vi "Sub Super Duper_2014 05 30_JWa.vi"(0 "VISA resource name":refnum<visa-resource-name>="GPIB0::17::INSTR", 1 "Sample Properties:":T9 {"Date Created" format="%<%Y/%m/%d>T"}, 2 "Gated SMU4 is...":bool, 3 "TRF Cluster":T10={"Step 4"=-38.0, "# of Loops"=1.0, "Transfer 2"=FALSE, "Start 4"=-2.0, "Total Points 2"=2, "Start 3"=40.0, "Stop 2"=-40.0, "Step 3"=-1.0, "Loop Step"=0.0, "Integration Time 3"=0, "Loop Wait"=0.0, "First Step"=0.0} {"Loop Wait" format="%<%H:%M:%S>t"; "Integration Time 3" scale=0.0..2.0; "Step 3" format="%.2f"; "Stop 2" format="%.2f"; "Start 3" format="%.2f"; "Start 4" format="%.2f"; "Step 4" format="%.2f"}, 4 "TSP Cluster":T11={"Transport"=FALSE, "Start 2"=0.0, "Stop 3"=-60.0, "Step 2"=-1.0, "Start"=0.0, "Step"=-10.0, "Total Points"=7, "Integration Time"=0} {"Integration Time" scale=0.0..2.0; "Step" format="%.2f"; "Start" format="%.2f"; "Step 2" format="%.2f"; "Stop 3" format="%.2f"; "Start 2" format="%.2f"}, 5 "Compliance Cluster":T6={"Var1 sweep settings"={"sweep spacing (linear: 0)"=0, "sweep mode"=FALSE, "compliance (V)"=100.0, "compliance (A)"=0.001}, "Var1 sweep settings 2"={"sweep spacing (linear: 0)"=0, "sweep mode"=FALSE, "compliance (V)"=100.0, "compliance (A)"=0.001}, "Var2 step settings 2"={"compliance (A)"=0.001, "compliance (V)"=100.0}, "Var2 step settings"={"compliance (A)"=0.001, "compliance (V)"=100.0}} {"Var2 step settings"."compliance (V)" format="%.2f"; "Var2 step settings"."compliance (A)" format="%^.2e"; "Var2 step settings 2"."compliance (V)" format="%.2f"; "Var2 step settings 2"."compliance (A)" format="%^.2e"; "Var1 sweep settings 2"."compliance (A)" format="%^.2e"; "Var1 sweep settings 2"."compliance (V)" format="%.2f"; "Var1 sweep settings 2"."sweep spacing (linear: 0)" items=["linear", "log 10", "log 25", "log 50"]; "Var1 sweep settings"."compliance (A)" format="%^.2e"; "Var1 sweep settings"."compliance (V)" format="%.2f"; "Var1 sweep settings"."sweep spacing (linear: 0)" items=["linear", "log 10", "log 25", "log 50"]}, 6 "Light Bathe Cluster":T2={"TG to BG:  "=FALSE, "TG to BG Durration"=120.0, "TRF to TSP:   "=FALSE, "TRF to TSP Duration"=120.0, "Post Measure: "=FALSE, "TG to BG (TSP):"=FALSE, "TG to BG Durration 3"=120.0} {"TG to BG Durration 3" format="%<%H:%M:%S>t"; "TRF to TSP Duration" format="%<%H:%M:%S>t"; "TG to BG Durration" format="%<%H:%M:%S>t"}, 7 "error in":errorcluster, 8 "Saved Folder:":path=path "C:/1DATA/2011", 9 "Wait Cluster":T5 {"Wait Time (s)" format="%.1g"; "Wait Countdown" format="%<%H:%M:%S%1u>t"}, 11 "TG Dielectric Prop":T1, 13 "Stop \nCountdown":bool, 15 "Loop Count":dbl, 16 "Gate Current Cluster":T3={"Gate Current (TSP)"={"Y2 axis on/off"=FALSE, "MINIMUM"=0.0, "MAXIMUM"=1.0, "Variable name"="Ig", "LIN or LOG axis"="LIN"}, "Gate Current (TRF)"={"Y2 axis on/off"=FALSE, "MINIMUM"=0.0, "MAXIMUM"=1.0, "Variable name"="Ig", "LIN or LOG axis"="LIN"}} {"Gate Current (TSP)"."MAXIMUM" format="%.9f"; "Gate Current (TSP)"."MINIMUM" format="%.9f"; "Gate Current (TRF)"."MAXIMUM" format="%.9f"; "Gate Current (TRF)"."MINIMUM" format="%.9f"}, 17 "Dielectric Constant (BG)":dbl) -> (12 "Status Indicator":bool, 14 "Vt Cluster":T4 {"Id Max" format="%.3g"; "Vt Max" format="%.3g"; "Vt Min" format="%.3g"; "Vt Ratio" format="%.3g"}, 20 "VISA resource name out":refnum<visa-resource-name>, 21 "TRF Path":path, 23 "TSP Path":path, 24 "Graph Cluster":T7, 25 "Char Cluster":T8 {"Mobility-Lin" format="%#_4e"; "On/Off" format="%#_4e"; "Mobility-Sat" format="%#_4e"}, 27 "error out":errorcluster)   [LabVIEW 2012]
uses:
  <vilib>/Platform/TimedLoop/XDataNode/wakeup.ctl
  <vilib>/Platform/TimedLoop/XDataNode/XDNodeRunTimeDep.lvlib
  <vilib>/Platform/TimedLoop/XDataNode/nitl_modes.ctl
  <vilib>/Platform/TimedLoop/XDataNode/timing_clust.ctl
  <vilib>/Platform/TimedLoop/XDataNode/XDataNode.xnode
panel:
  in  "Ambient Temp (Y/N)":bool=TRUE
  out "LKG Path":path
  # "Vg Sweep"
  # "Vd Step"
  # "Loops and Integration Time"
  # "Device Characteristics"
  # "Light Bath is..."
  # "Duration (hh:mm:ss)"
  # "Sample Properties:"
  # "%"
  # "nm"
  # "Device Properties:"
  # "um"
  # "um"
  # "Vg Step"
  # "Vd Step"
  # "Integration Time"
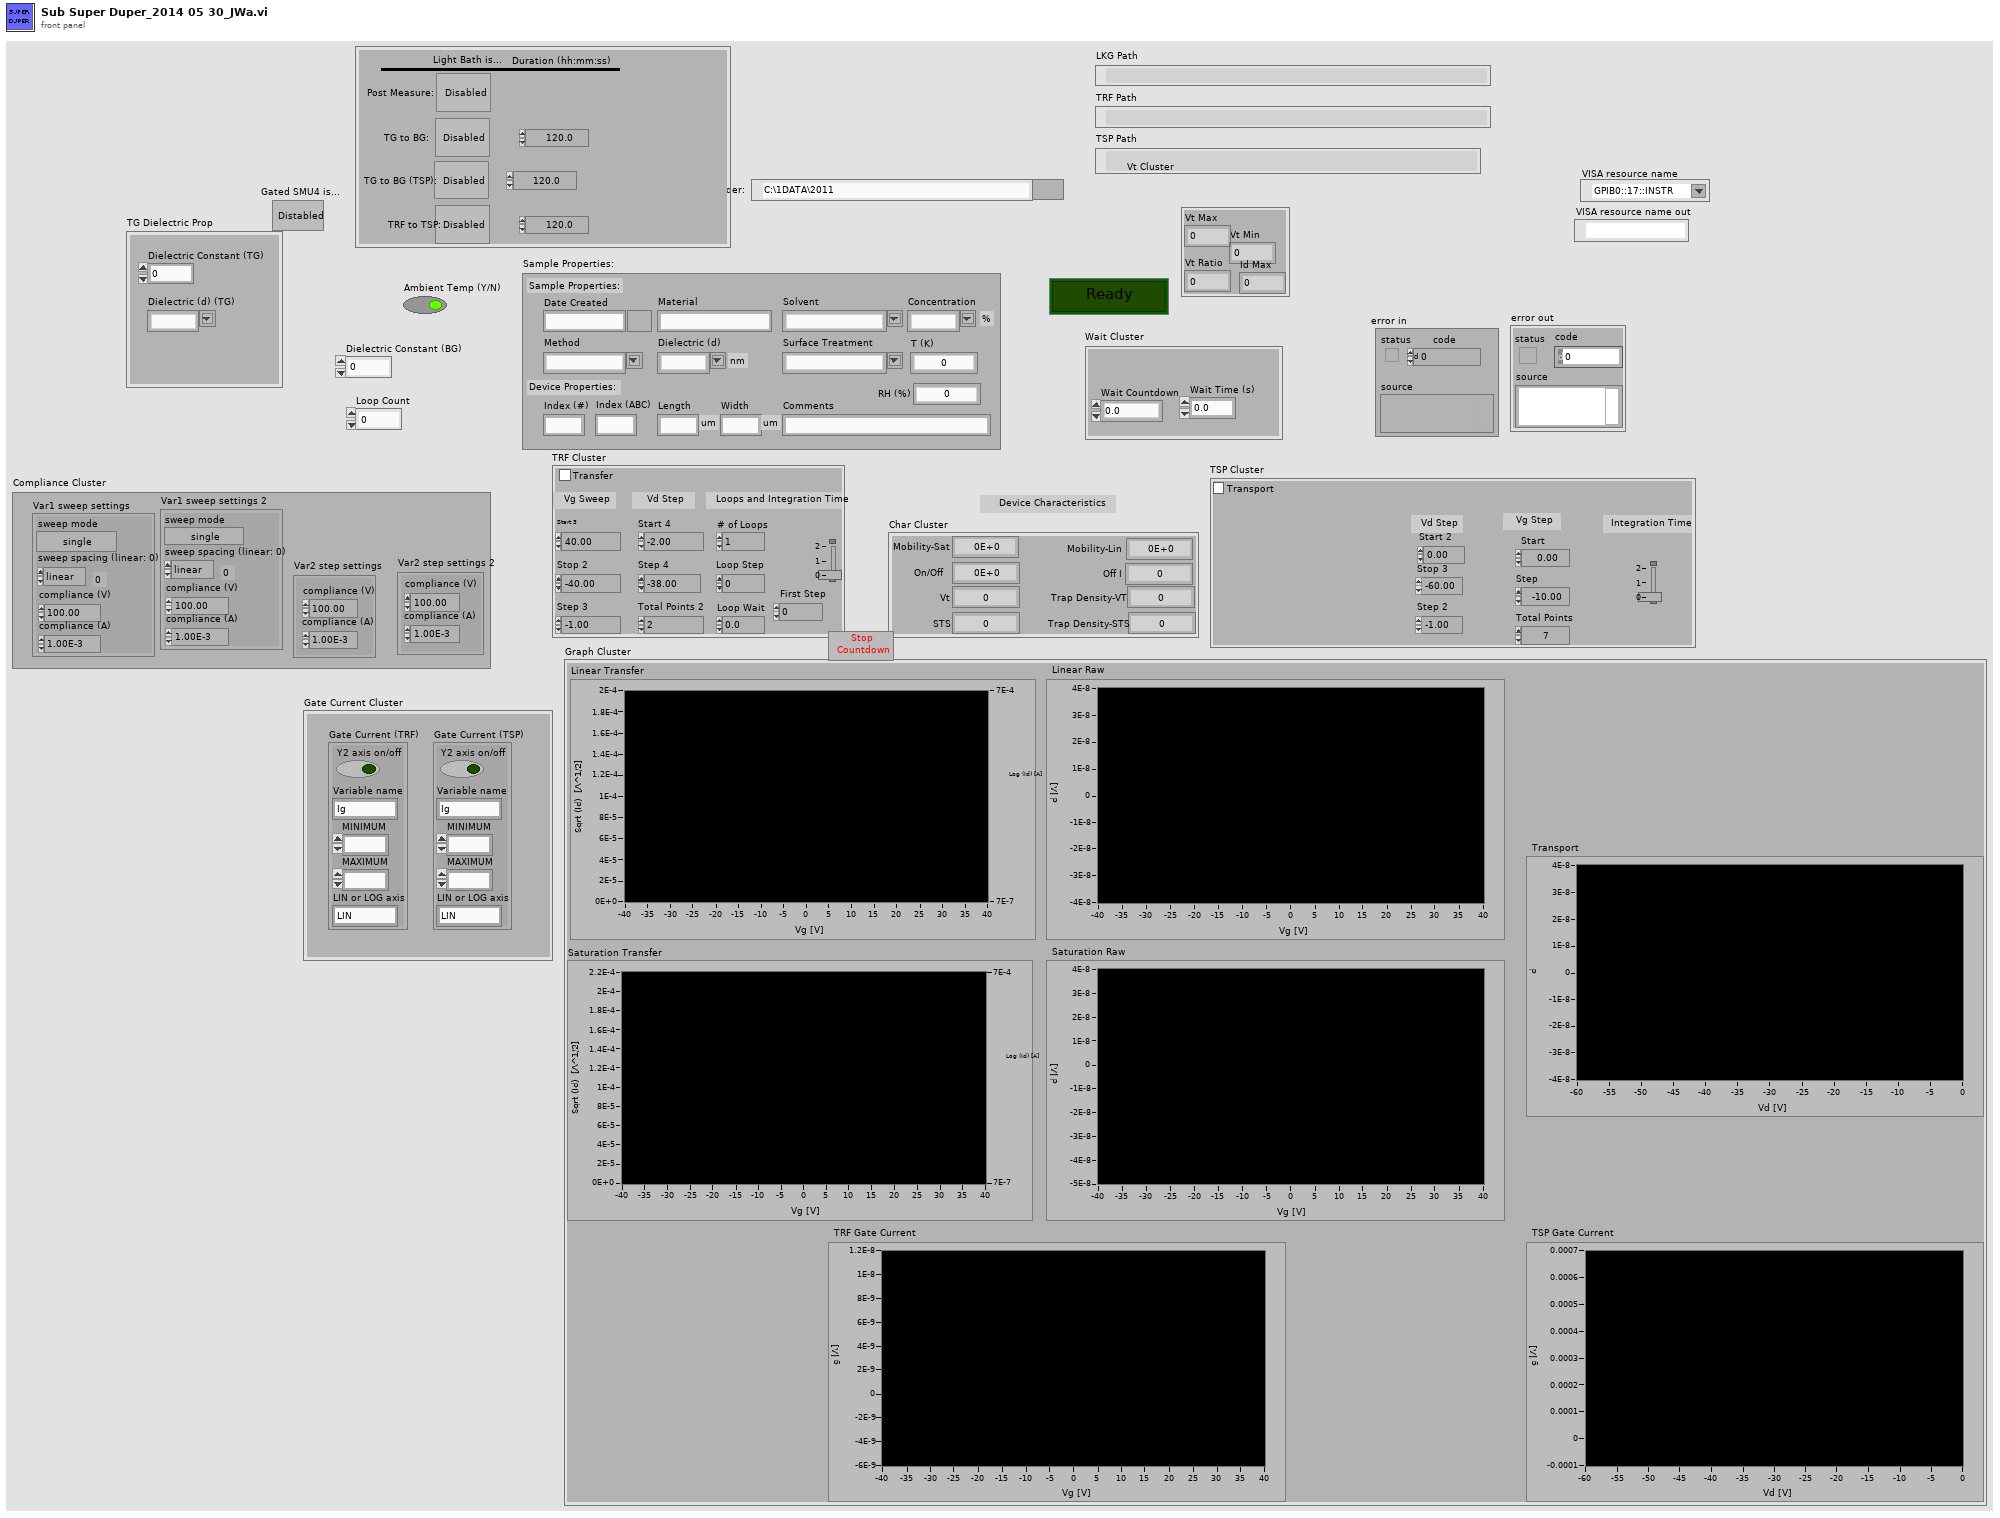
[diagram p1: front panel]
types:
  T1 = cluster{"Dielectric Constant (TG)":dbl, "Dielectric (d) (TG)":string}
  T2 = cluster{"TG to BG:  ":bool, "TG to BG Durration":dbl, "TRF to TSP:   ":bool, "TRF to TSP Duration":dbl, "Post Measure: ":bool, "TG to BG (TSP):":bool, "TG to BG Durration 3":dbl}
  T3 = cluster{"Gate Current (TSP)":cluster{"Y2 axis on/off":bool, "MINIMUM":ext, "MAXIMUM":ext, "Variable name":string, "LIN or LOG axis":string}, "Gate Current (TRF)":cluster{"Y2 axis on/off":bool, "MINIMUM":ext, "MAXIMUM":ext, "Variable name":string, "LIN or LOG axis":string}}
  T4 = cluster{"Vt Max":i32, "Vt Min":i32, "Vt Ratio":i32, "Id Max":i32}
  T5 = cluster{"Wait Countdown":dbl, "Wait Time (s)":dbl}
  T6 = cluster{"Var1 sweep settings":cluster{"sweep spacing (linear: 0)":u16, "sweep mode":bool, "compliance (V)":dbl, "compliance (A)":dbl}, "Var1 sweep settings 2":cluster{"sweep spacing (linear: 0)":u16, "sweep mode":bool, "compliance (V)":dbl, "compliance (A)":dbl}, "Var2 step settings 2":cluster{"compliance (A)":dbl, "compliance (V)":dbl}, "Var2 step settings":cluster{"compliance (A)":dbl, "compliance (V)":dbl}}
  T7 = cluster{"Linear Transfer":cluster{dbl[], "trace":dbl[]}[], "Linear Raw":cluster{dbl[], dbl[]}[], "Saturation Transfer":cluster{dbl[], "trace":dbl[]}[], "Saturation Raw":cluster{dbl[], dbl[]}[], "Transport":cluster{dbl[], dbl[]}[], "TRF Gate Current":cluster{dbl[], dbl[]}[], "TSP Gate Current":cluster{dbl[], dbl[]}[]}
  T8 = cluster{"Mobility-Sat":dbl, "Mobility-Lin":dbl, "On/Off ":dbl, "Off I":dbl, "Vt":dbl, "STS":dbl, "Trap Density-VT":dbl, "Trap Density-STS":dbl}
  T9 = cluster{"Date Created":timestamp, "Material":string, "Solvent":string, "Concentration":string, "Method":string, "Dielectric (d)":string, "Index (#)":string, "Index (ABC)":string, "Length":string, "Width":string, "Surface Treatment":string, "Comments":string, "T (K)":dbl, "RH (%)":dbl}
  T10 = cluster{"Step 4":dbl, "# of Loops":dbl, "Transfer 2":bool, "Start 4":dbl, "Total Points 2":u16, "Start 3":dbl, "Stop 2":dbl, "Step 3":dbl, "Loop Step":dbl, "Integration Time 3":u32, "Loop Wait":dbl, "First Step":dbl}
  T11 = cluster{"Transport":bool, "Start 2":dbl, "Stop 3":dbl, "Step 2":dbl, "Start":dbl, "Step":dbl, "Total Points":u16, "Integration Time":u32}
  T12 = cluster{"Vname":string, "Vname 2":string, "Vname 3":string, "Vname 4":string, "Iname":string, "Iname 2":string, "Iname 3":string, "Iname 4":string, "Mode":u16, "Mode 2":u16, "Mode 3":u16, "Mode 4":u16, "Function":u16, "Function 2":u16, "Function 3":u16, "Function 4":u16, "Value (V or A)":dbl, "Value (Either V or A) 2":dbl, "Value (Either V or A) 3":dbl, "Value (Either V or A) 4":dbl}
  T13 = typedef "XDNodeRunTimeDep.lvlib/timing_clust.ctl" = cluster{"Expected End [f-1]":u64, "Actual End [f-1]":u64, "Finished Late? [f-1]":bool, "Expected End [i-1]":u64, "Actual End [i-1]":u64, "Finished Late? [i-1]":bool, "Expected Start [i]":u64, "Actual Start [i]":u64, "Expected Start [f]":u64, "Actual Start [f]":u64, "Source Name":string, "Structure Name":string, "Period":i64, "Deadline":i64, "Offset":i64, "Start":i64, "Priority":i32, "Timeout":i32, "Mode":T14, "Wakeup Reason":T15, "Error":errorcluster, "Source Type":string, "Secondary Source Type":string, "Global End Time":u64, "Global Start Time":u64, "Frame Duration":u64, "Iteration Duration":u64, "Assigned CPU":i32, "I/O Scan Engine Mode":u32}
  T14 = typedef "XDNodeRunTimeDep.lvlib/nitl_modes.ctl" = enum32{"No Change", "Process missed periods, maintain original phase", "Discard missed periods, maintain original phase", "Process missed periods, ignore original phase", "Discard missed periods, ignore original phase"}
  T15 = typedef "XDNodeRunTimeDep.lvlib/wakeup.ctl" = enum32{"Normal", "Aborted", "Asynchronous wakeup", "Timing source error", "Timed loop error", "Timeout"}
  T16 = cluster{"sweep spacing (linear: 0)":u16, "sweep mode":bool, "compliance (V)":dbl, "compliance (A)":dbl}
  T17 = cluster{"compliance (A)":dbl, "compliance (V)":dbl}
  T18 = cluster{"Y2 axis on/off":bool, "MINIMUM":ext, "MAXIMUM":ext, "Variable name":string, "LIN or LOG axis":string}
  T19 = cluster{"Start 3":dbl, "Stop 2":dbl, "Step 3":dbl, "sweep spacing (linear: 0)":u16, "sweep mode":bool, "compliance (V)":dbl, "compliance (A)":dbl}
  T20 = cluster{"compliance (A)":dbl, "compliance (V)":dbl, "Start 4":dbl, "Total Points 2":u16, dbl}
  T21 = cluster{"Vt Max":i32, "Vt Min":i32, "Vt Ratio":i32, "Id Max":dbl}
  T22 = cluster{"Mobility-Sat":dbl, "Mobility-Lin":dbl, "On/Off Current":dbl, "Off I":dbl, "Vt":dbl, "STS":dbl, "Trap Density-VT":dbl, "Trap Density-STS":dbl}
  T23 = cluster{"Linear Sqrt":cluster{dbl[], "trace":dbl[]}[], "Linear Log":cluster{dbl[], "trace":dbl[]}[], "Linear Raw":cluster{dbl[], dbl[]}[], "Saturation Sqrt":cluster{dbl[], "trace":dbl[]}[], "Saturation Log":cluster{dbl[], "trace":dbl[]}[], "Saturation Raw":cluster{dbl[], "trace":dbl[]}[], "Gate Current":cluster{dbl[], "trace":dbl[]}[]}
  T24 = cluster{"Start 2":dbl, "Stop 3":dbl, "Step 2":dbl, "sweep spacing (linear: 0)":u16, "sweep mode":bool, "compliance (V)":dbl, "compliance (A)":dbl}
  T25 = cluster{"compliance (A)":dbl, "compliance (V)":dbl, "Start":dbl, "Total Points":u16, "Step":dbl}
  T26 = cluster{"Transport":cluster{dbl[], dbl[]}[], "Gate Current":cluster{dbl[], dbl[]}[]}
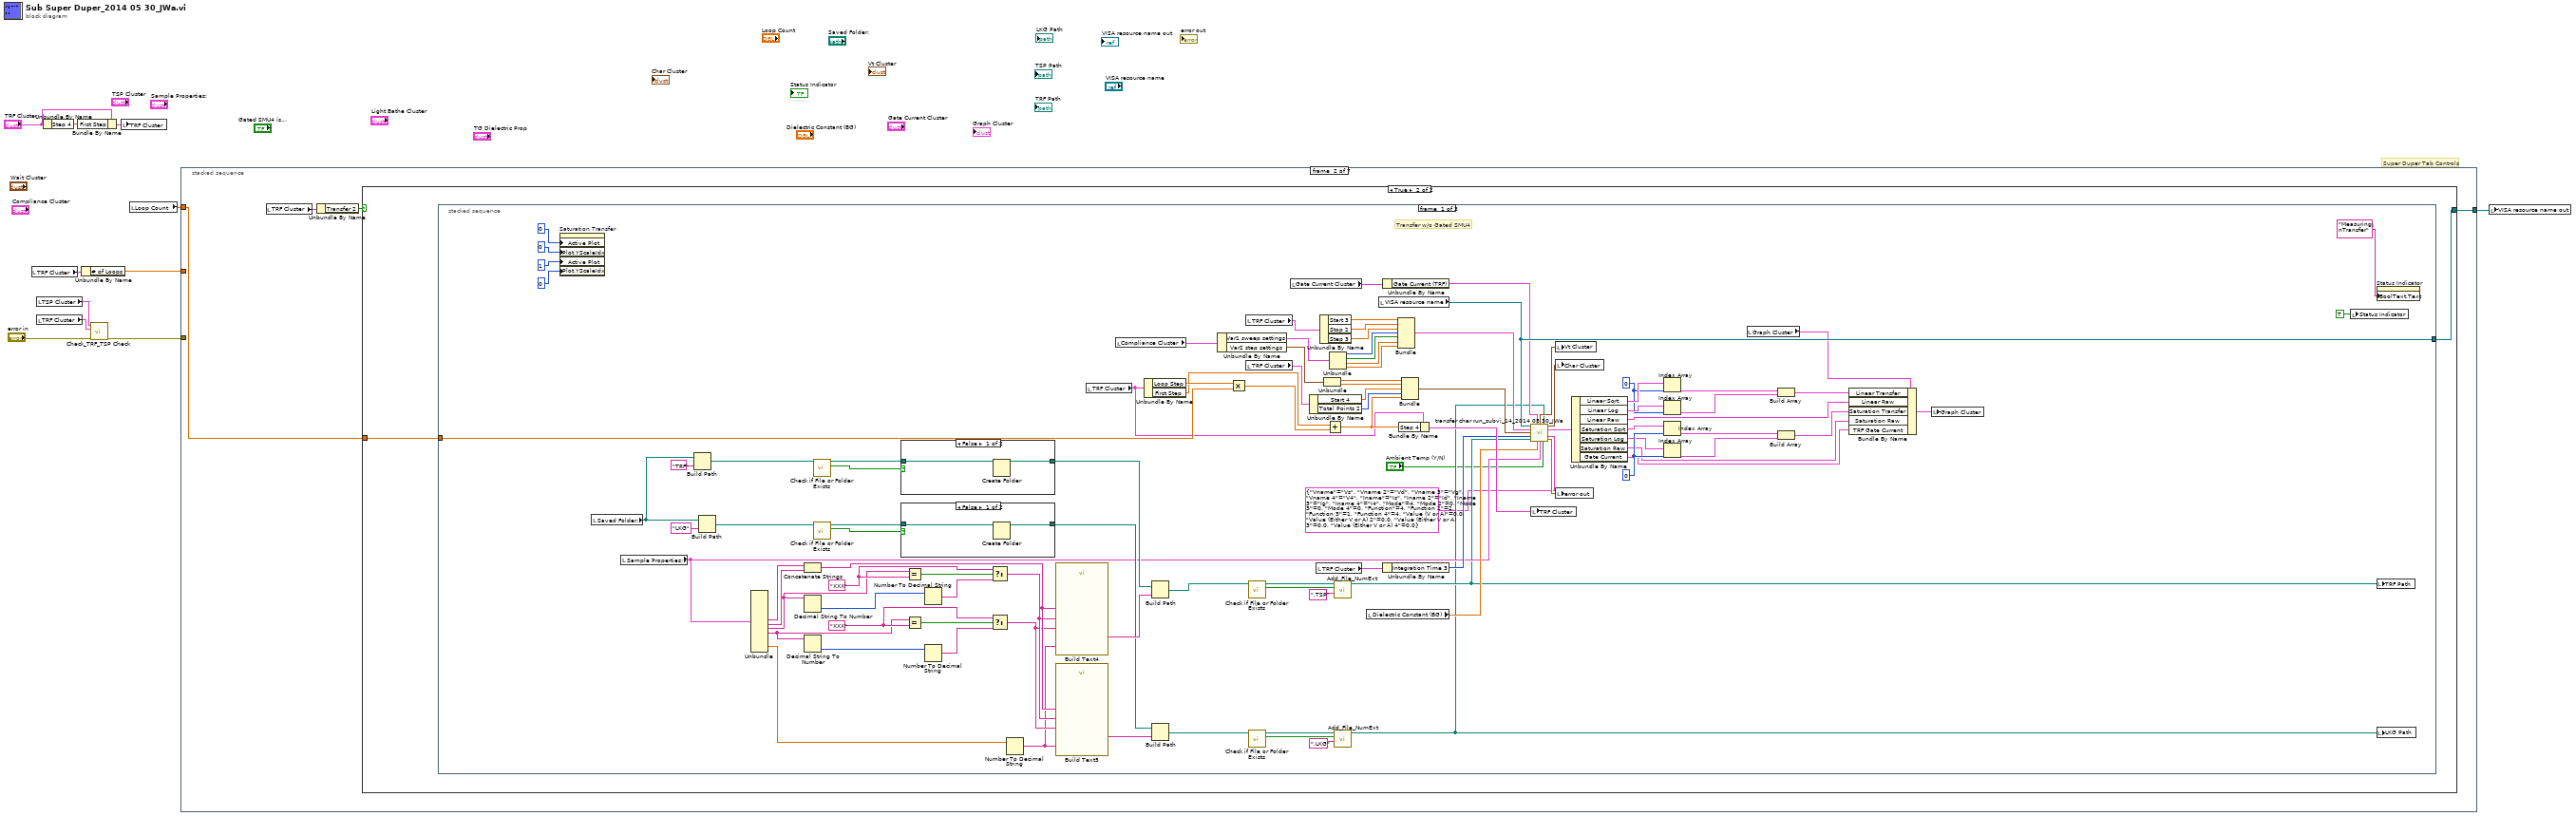
[diagram p0: block diagram]
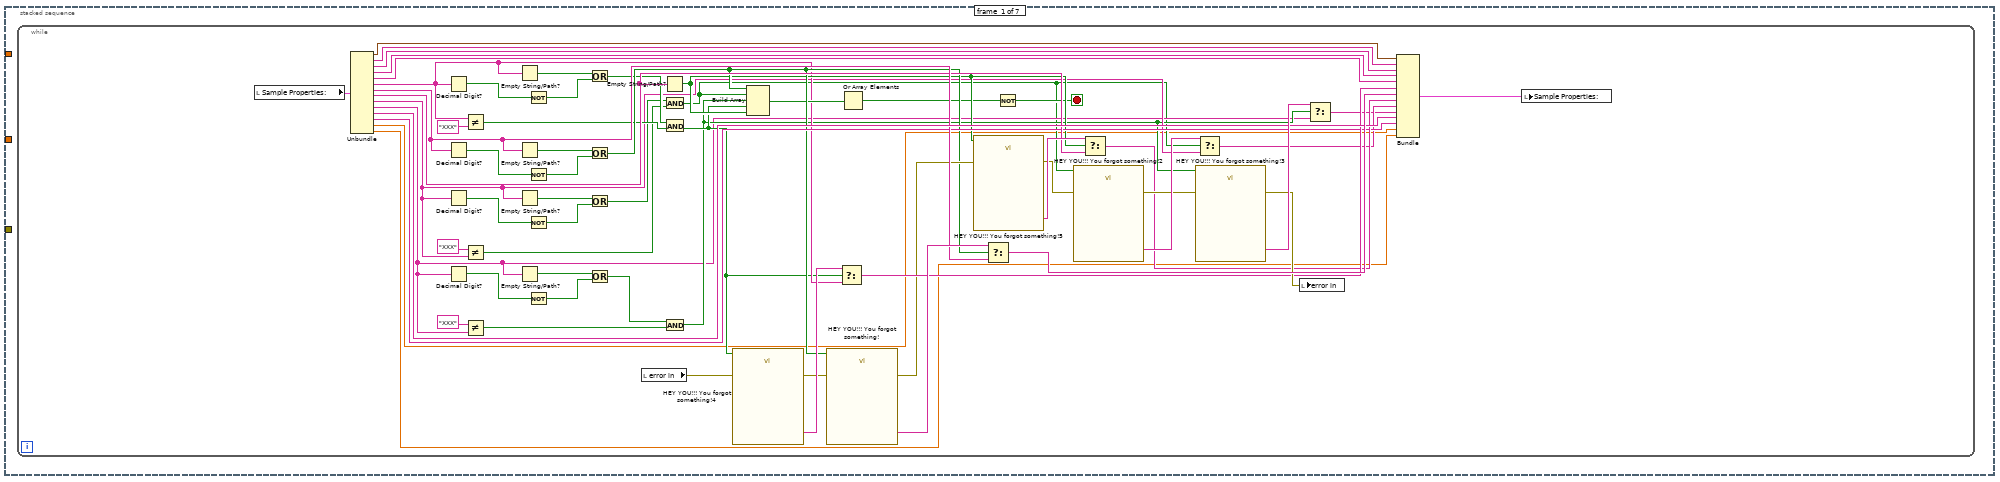
[diagram p2: hidden frame]
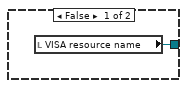
[diagram p3: hidden frame]
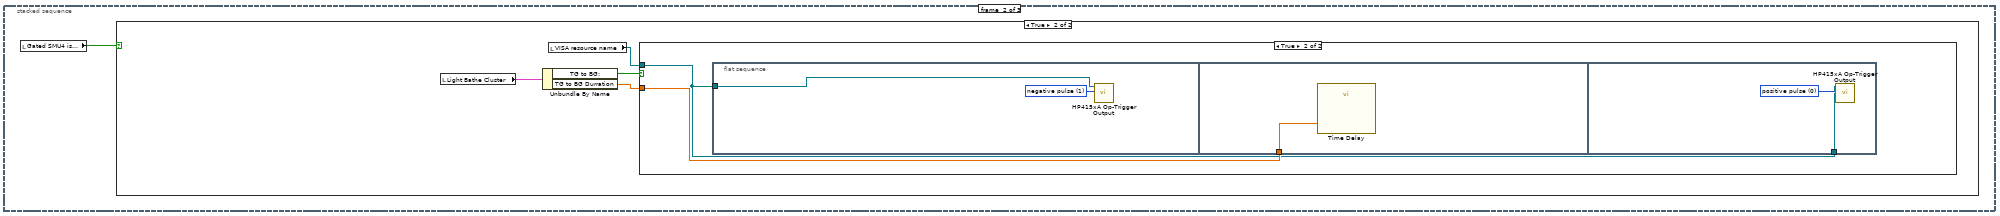
[diagram p6: hidden frame]
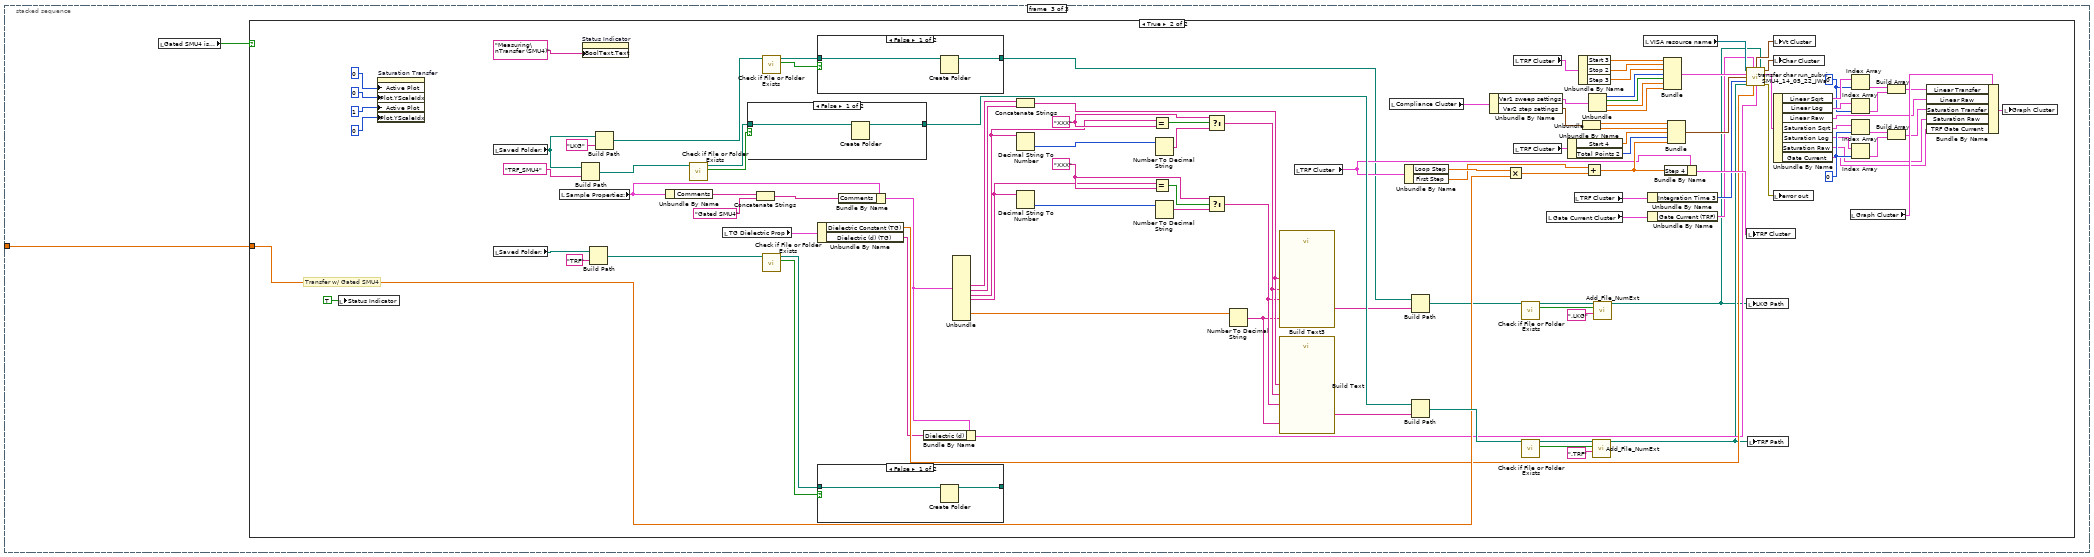
[diagram p9: hidden frame]
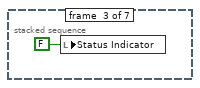
[diagram p14: hidden frame]
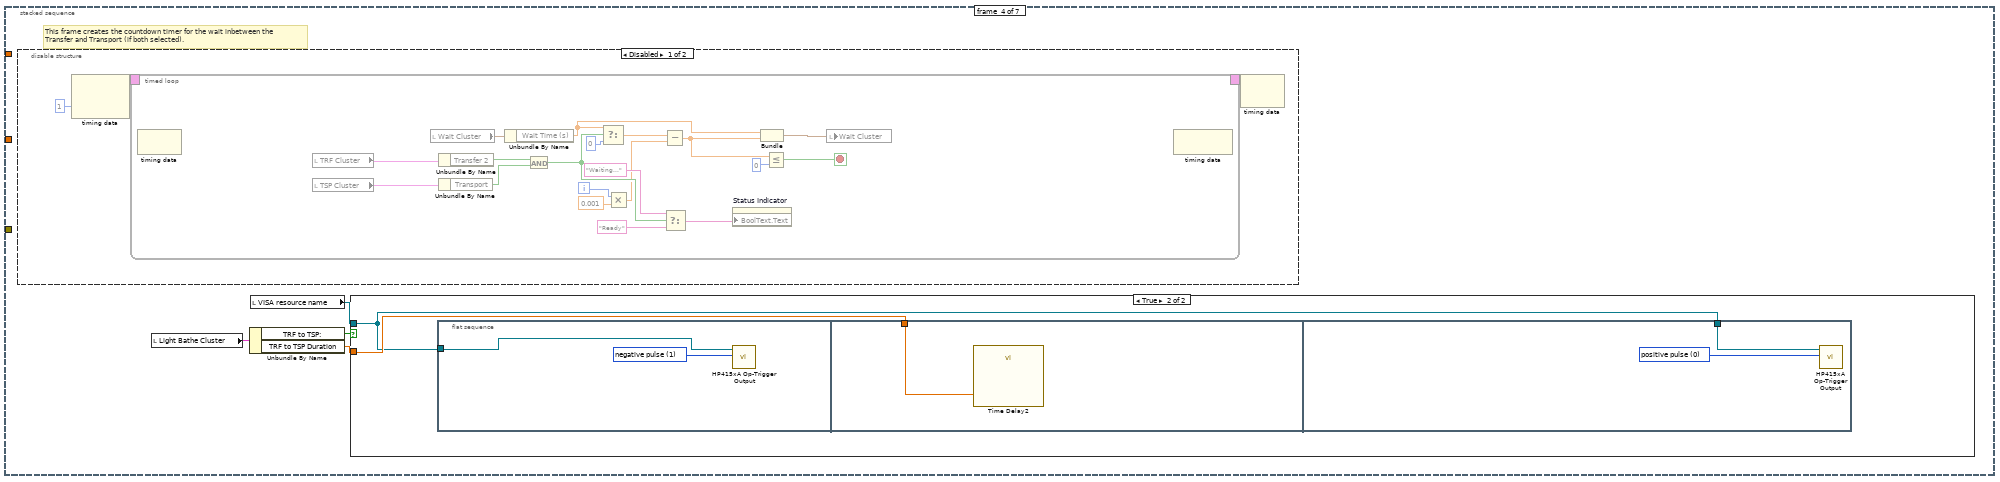
[diagram p15: hidden frame]
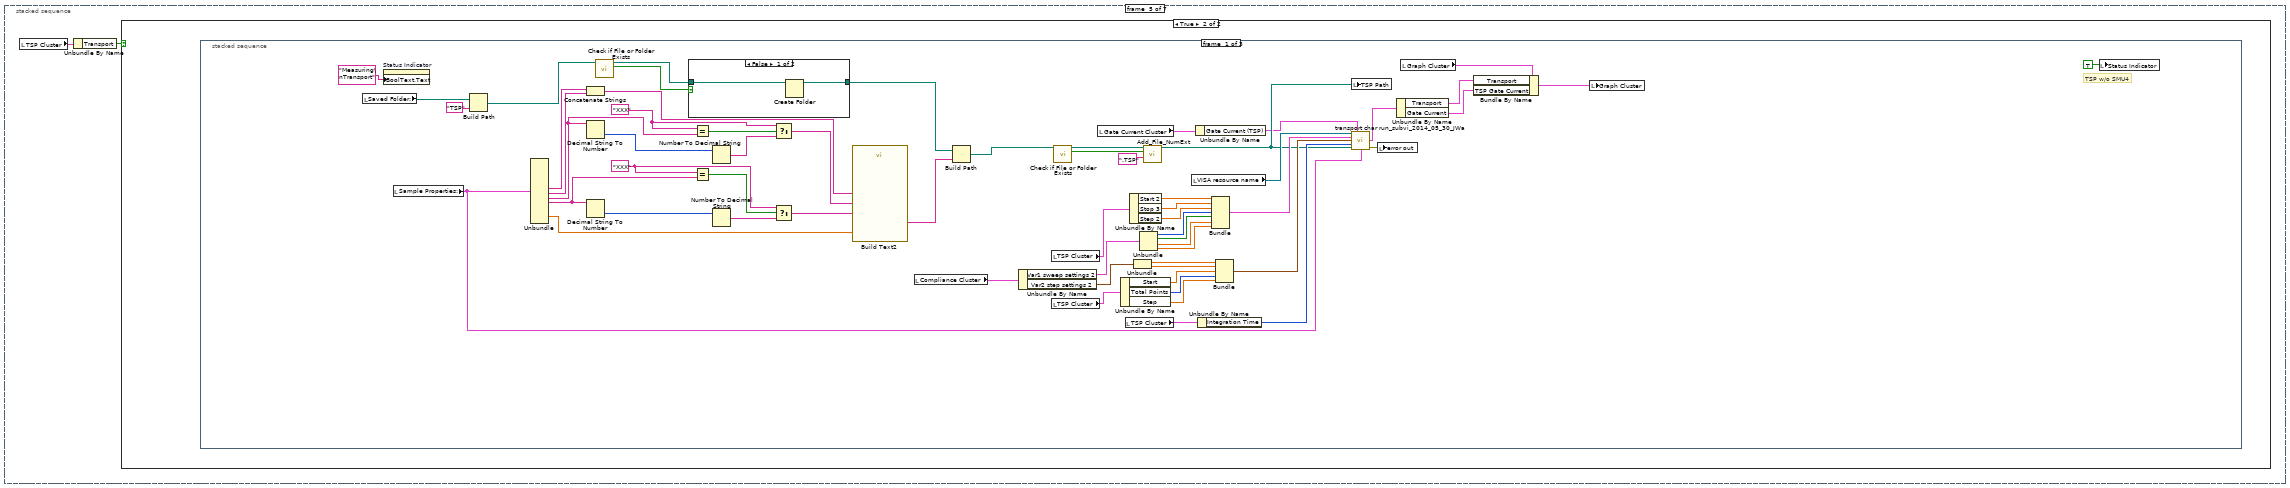
[diagram p18: hidden frame]
diagram:
  # "Super Duper Tab Controls"
  n1 = local read "TRF Cluster"() -> (w8:T10)
  n2 = local read "TSP Cluster"() -> (w4:T11)
  n3 = local read "TRF Cluster"() -> (w3:T10)
  n4 = Unbundle By Name("TRF Cluster") -> ("Step 4"=w9:dbl)
  n5 = Bundle By Name(cluster="TRF Cluster", "First Step"=w9) -> (w11:T10)
  n6 = Unbundle By Name(w8) -> ("# of Loops"=w7:dbl)
  n7 = call "Check_TRF_TSP Check.vi"("error in"="error in", "TRF Cluster"=w3, "TSP Cluster"=w4) -> ("error out"=w1:errorcluster)  [unwired: 8 in]
  n8 = local write "TRF Cluster"(w11) -> ()
  n9 = local read "Loop Count"() -> (w5:dbl)
  n10 = stacked-sequence {
    tunnel: w5 -> [_ w76 _ _ _ _ w507]
    tunnel: w7 -> [_ _ _ _ _ _ w506]
    tunnel: [_ w73 _ _ _ _ _] -> w6
    tunnel: w1 -> [_ _ _ _ _ _ _]
    frame #0 {
      n11 = while {
        stop <- w38 stop-if-true
        n12 = local read "Sample Properties:"() -> (w67:T9)
        n13 = Unbundle(w67) -> ("Date Created"=w68:timestamp, "Material"=w69:string, "Solvent"=w70:string, "Concentration"=w71:string, "Method"=w72:string, "Dielectric (d)"=w27:string, "Index (#)"=w57:string, "Index (ABC)"=w54:string, "Length"=w22:string, "Width"=w15:string, "Surface Treatment"=w60:string, "Comments"=w52:string, "T (K)"=w13:dbl, "RH (%)"=w12:dbl)
        n14 = Decimal Digit?(1:w27) -> (0:w35:bool)
        n15 = Decimal Digit?(1:w57) -> (0:w48:bool)
        n16 = Decimal Digit?(1:w22) -> (0:w37:bool)
        n17 = Decimal Digit?(1:w15) -> (0:w36:bool)
        n18 = Not Equal?(x=w27, y="XXX") -> (x != y?=w26:bool)
        n19 = Not Equal?(x="XXX", y=w22) -> (x != y?=w21:bool)
        n20 = Not Equal?(x="XXX", y=w15) -> (x != y?=w19:bool)
        n21 = Empty String/Path?(string/path=w27) -> (empty?=w29:bool)
        n22 = Empty String/Path?(string/path=w57) -> (empty?=w56:bool)
        n23 = Empty String/Path?(string/path=w22) -> (empty?=w31:bool)
        n24 = Empty String/Path?(string/path=w15) -> (empty?=w30:bool)
        n25 = Not(x=w35) -> (.not. x?=w32:bool)
        n26 = Not(x=w48) -> (.not. x?=w47:bool)
        n27 = Not(x=w37) -> (.not. x?=w34:bool)
        n28 = Not(x=w36) -> (.not. x?=w33:bool)
        n29 = Or(x=w29, y=w32) -> (x .or. y?=w25:bool)
        n30 = Or(x=w56, y=w47) -> (x .or. y?=w42:bool)
        n31 = Or(x=w31, y=w34) -> (x .or. y?=w20:bool)
        n32 = Or(x=w30, y=w33) -> (x .or. y?=w18:bool)
        n33 = local read "error in"() -> (w44:errorcluster)
        n34 = Empty String/Path?(string/path=w54) -> (empty?=w41:bool)
        n35 = And(x=w20, y=w21) -> (x .and. y?=w14:bool)
        n36 = And(x=w25, y=w26) -> (x .and. y?=w24:bool)
        n37 = And(x=w18, y=w19) -> (x .and. y?=w17:bool)
        n38 = call "HEY YOU!!! You forgot something!4"("Enable"=w24, "error in (no error)"=w44) -> ("Dielectric (d)"=w59:string, "error out"=w43:errorcluster)  [unwired: 15 in, 1 out]
        n39 = Build Array(w42, w14, w17, w24, w41) -> (w40:bool[])
        n40 = call "HEY YOU!!! You forgot something!"("Enable"=w42, "error in (no error)"=w43) -> ("Index (#)"=w66:string, "error out"=w46:errorcluster)  [unwired: 15 in, 1 out]
        n41 = Select(t=w59, s=w24, f=w27) -> (s? t:f=w58:string)
        n42 = Or Array Elements(Boolean array=w40) -> (logical OR=w39:bool)
        n43 = call "HEY YOU!!! You forgot something!5"("Enable"=w41, "error in (no error)"=w46) -> ("Index (ABC)"=w55:string, "error out"=w45:errorcluster)  [unwired: 15 in, 1 out]
        n44 = Select(t=w66, s=w42, f=w57) -> (s? t:f=w63:string)
        n45 = Not(x=w39) -> (.not. x?=w38:bool)
        n46 = call "HEY YOU!!! You forgot something!2"("Enable"=w14, "error in (no error)"=w45) -> ("Length"=w65:string, "error out"=w62:errorcluster)  [unwired: 15 in, 1 out]
        n47 = Select(t=w55, s=w41, f=w54) -> (s? t:f=w53:string)
        n48 = call "HEY YOU!!! You forgot something!3"("Enable"=w17, "error in (no error)"=w62) -> ("Width"=w64:string, "error out"=w61:errorcluster)  [unwired: 15 in, 1 out]
        n49 = Select(t=w65, s=w14, f=w22) -> (s? t:f=w51:string)
        n50 = local write "error in"(w61) -> ()
        n51 = Select(t=w64, s=w17, f=w15) -> (s? t:f=w50:string)
        n52 = Bundle("Date Created"=w68, "Material"=w69, "Solvent"=w70, "Concentration"=w71, "Method"=w72, "Dielectric (d)"=w58, "Index (#)"=w63, "Index (ABC)"=w53, "Length"=w51, "Width"=w50, "Surface Treatment"=w60, "Comments"=w52, "T (K)"=w13, "RH (%)"=w12) -> (w49:T9)  [unwired: 1 in]
        n53 = local write "Sample Properties:"(w49) -> ()
      }
    }
    frame #1 {
      n54 = local read "TRF Cluster"() -> (w74:T10)
      n55 = Unbundle By Name(w74) -> ("Transfer 2"=w75:bool)
      n56 = case shown="True" w75 {
        tunnel: w76 -> [_ w79]
        tunnel: [w77 w78] -> w73
        frame False {
          n57 = local read "VISA resource name"() -> (w77:refnum<visa-resource-name>)
        }
        frame True {
          n58 = stacked-sequence {
            tunnel: w79 -> [w180 _ w200]
            tunnel: [w179 _ _] -> w78
            frame #0 {
              w113 = 0
              w119 = 0
              w160 = "XXX"
              w163 = "XXX"
              # "Transfer w/o Gated SMU4"
              n59 = property on="Saturation Transfer" class="XYGraph (strict)"("Active Plot"=0, "Plot.YScaleIdx"=0, "Active Plot"=1, "Plot.YScaleIdx"=0) -> ()  [unwired: 2 in, 2 out]
              n60 = local read "Saved Folder:"() -> (w105:path)
              n61 = local read "Sample Properties:"() -> (w90:T9)
              n62 = Build Path(base path=w105, name or relative path="TRF") -> (appended path=w153:path)
              n63 = Build Path(base path=w105, name or relative path="LKG") -> (appended path=w101:path)
              n64 = Unbundle(w90) -> ("Index (#)"=w169:string, "Index (ABC)"=w168:string, "Length"=w157:string, "Width"=w159:string, "T (K)"=w136:dbl)  [unwired: 9 out]
              n65 = Concatenate Strings(w169, w168) -> (w98:string)
              n66 = Decimal String To Number(string=w157) -> (number=w166:i32)  [unwired: 2 in, 1 out]
              n67 = Decimal String To Number(string=w159) -> (number=w165:i32)  [unwired: 2 in, 1 out]
              n68 = call <vilib>:"Check if File or Folder Exists.vi"("path"=w153) -> ("file or folder exists?"=w155:bool, "dup path"=w154:path)  [unwired: 8 in, 1 out]
              n69 = call <vilib>:"Check if File or Folder Exists.vi"("path"=w101) -> ("file or folder exists?"=w102:bool, "dup path"=w103:path)  [unwired: 8 in, 1 out]
              n70 = case shown="False" w155 {
                tunnel: w154 -> [w185 w186]
                tunnel: [w184 w186] -> w152
                frame False {
                  n71 = Create Folder(path (use dialog)=w185) -> (created path=w184:path)  [unwired: 2 in, 2 out]
                }
                frame True {
                }
              }
              n72 = case shown="False" w102 {
                tunnel: w103 -> [w182 w183]
                tunnel: [w181 w183] -> w94
                frame False {
                  n73 = Create Folder(path (use dialog)=w182) -> (created path=w181:path)  [unwired: 2 in, 2 out]
                }
                frame True {
                }
              }
              n74 = Equal?(x=w157, y=w163) -> (x = y?=w164:bool)
              n75 = Equal?(x=w159, y=w160) -> (x = y?=w161:bool)
              n76 = Number To Decimal String(number=w166) -> (decimal integer string=w162:string)  [unwired: 1 in]
              n77 = Number To Decimal String(number=w165) -> (decimal integer string=w158:string)  [unwired: 1 in]
              n78 = Select(t=w163, s=w164, f=w162) -> (s? t:f=w97:string)
              n79 = Select(t=w160, s=w161, f=w158) -> (s? t:f=w96:string)
              n80 = Number To Decimal String(number=w136) -> (decimal integer string=w95:string)  [unwired: 1 in]
              n81 = call "Build Text4"("T"=w95, "Index"=w98, "Length"=w97, "Width"=w96) -> ("Result"=w172:string)  [unwired: 10 in, 1 out]
              n82 = call "Build Text5"("T"=w95, "Index"=w98, "Length"=w97, "Width"=w96) -> ("Result"=w99:string)  [unwired: 10 in, 1 out]
              n83 = local read "TRF Cluster"() -> (w130:T10)
              n84 = local read "Compliance Cluster"() -> (w139:T6)
              n85 = Unbundle By Name(w130) -> ("Loop Step"=w133:dbl, "First Step"=w132:dbl)
              n86 = Build Path(base path=w152, name or relative path=w172) -> (appended path=w167:path)
              n87 = Build Path(base path=w94, name or relative path=w99) -> (appended path=w100:path)
              n88 = Unbundle By Name(w139) -> ("Var1 sweep settings"=w137:T16, "Var2 step settings"=w138:T17)
              n89 = Multiply(x=w133, y=w180) -> (x*y=w135:dbl)
              n90 = local read "TRF Cluster"() -> (w144:T10)
              n91 = local read "TRF Cluster"() -> (w147:T10)
              n92 = call <vilib>:"Check if File or Folder Exists.vi"("path"=w167) -> ("file or folder exists?"=w87:bool, "dup path"=w86:path)  [unwired: 8 in, 1 out]
              n93 = call <vilib>:"Check if File or Folder Exists.vi"("path"=w100) -> ("file or folder exists?"=w82:bool, "dup path"=w83:path)  [unwired: 8 in, 1 out]
              n94 = local read "Gate Current Cluster"() -> (w93:T3)
              n95 = Unbundle By Name(w147) -> ("Start 4"=w146:dbl, "Total Points 2"=w145:u16)
              n96 = local read "TRF Cluster"() -> (w140:T10)
              n97 = Unbundle By Name(w144) -> ("Start 3"=w143:dbl, "Stop 2"=w142:dbl, "Step 3"=w141:dbl)
              n98 = Unbundle(w138) -> ("compliance (A)"=w174:dbl, "compliance (V)"=w173:dbl)
              n99 = Add(x=w132, y=w135) -> (x+y=w131:dbl)
              n100 = Unbundle(w137) -> ("sweep spacing (linear: 0)"=w178:u16, "sweep mode"=w177:bool, "compliance (V)"=w176:dbl, "compliance (A)"=w175:dbl)
              n101 = call "Add_File_NumExt.vi"("Extension"=".TSP" ("string"), "file or folder exists?"=w87, "Path In"=w86) -> ("Path Out"=w89:path)  [unwired: 8 in]
              n102 = call "Add_File_NumExt.vi"("Extension"=".LKG" ("string"), "file or folder exists?"=w82, "Path In"=w83) -> ("Path Out"=w85:path)  [unwired: 8 in]
              n103 = local read "Dielectric Constant (BG)"() -> (w91:dbl)
              n104 = local read "VISA resource name"() -> (w179:refnum<visa-resource-name>)
              n105 = Unbundle By Name(w93) -> ("Gate Current (TRF)"=w92:T18)
              n106 = Unbundle By Name(w140) -> ("Integration Time 3"=w127:u32)
              n107 = Bundle("Start 3"=w143, "Stop 2"=w142, "Step 3"=w141, "sweep spacing (linear: 0)"=w178, "sweep mode"=w177, "compliance (V)"=w176, "compliance (A)"=w175) -> (w129:T19)  [unwired: 1 in]
              n108 = Bundle By Name(cluster=w130, "Step 4"=w131) -> (w134:T10)
              n109 = Bundle("compliance (A)"=w174, "compliance (V)"=w173, "Start 4"=w146, "Total Points 2"=w145, w131) -> (w128:T20)  [unwired: 1 in]
              n110 = call "transfer char run_subvi_14_2014 05 30_JWa.vi"("VISA session"=w179, "Y2 axis settings"=w92, "LKG Path"=w85, "Var1 sweep settings"=w129, "Var2 step settings"=w128, "integration time"=w127, "SMU Config"=T12 {"Vname"="Vs", "Vname 2"="Vd", "Vname 3"="Vg", "Vname 4"="V4", "Iname"="Is", "Iname 2"="Id", "Iname 3"="Ig", "Iname 4"="I4", "Mode"=4, "Mode 2"=0, "Mode 3"=0, "Mode 4"=0, "Function"=4, "Function 2"=2, "Function 3"=1, "Function 4"=4, "Value (V or A)"=0.0, "Value (Either V or A) 2"=0.0, "Value (Either V or A) 3"=0.0, "Value (Either V or A) 4"=0.0}, "Input Path"=w89, "Dielectric Constant"=w91, "Sample Properties:"=w90, "Ambient Temp (Y/N)"="Ambient Temp (Y/N)") -> ("Check Cluster"=w124:T21, "Output"=w125:T22, "Graph Cluster"=w123:T23, "Error In"=w126:errorcluster)  [unwired: 1 in]
              n111 = local write "TRF Cluster"(w134) -> ()
              n112 = local write "Vt Cluster"(w124) -> ()
              n113 = local write "Char Cluster"(w125) -> ()
              n114 = local write "error out"(w126) -> ()
              n115 = Unbundle By Name(w123) -> ("Linear Sqrt"=w121:cluster{dbl[], "trace":dbl[]}[], "Linear Log"=w120:cluster{dbl[], "trace":dbl[]}[], "Linear Raw"=w109:cluster{dbl[], dbl[]}[], "Saturation Sqrt"=w112:cluster{dbl[], "trace":dbl[]}[], "Saturation Log"=w111:cluster{dbl[], "trace":dbl[]}[], "Saturation Raw"=w108:cluster{dbl[], "trace":dbl[]}[], "Gate Current"=w106:cluster{dbl[], "trace":dbl[]}[])
              n116 = Index Array(array=w121, index=w119) -> (element=w118:cluster{dbl[], "trace":dbl[]})
              n117 = Index Array(array=w120, index=w119) -> (element=w117:cluster{dbl[], "trace":dbl[]})
              n118 = Index Array(array=w112, index=w113) -> (element=w114:cluster{dbl[], "trace":dbl[]})
              n119 = Index Array(array=w111, index=w113) -> (element=w115:cluster{dbl[], "trace":dbl[]})
              n120 = local read "Graph Cluster"() -> (w122:T7)
              n121 = Build Array(w118, w117) -> (w116:cluster{dbl[], "trace":dbl[]}[])
              n122 = Build Array(w114, w115) -> (w110:cluster{dbl[], "trace":dbl[]}[])
              n123 = Bundle By Name(cluster=w122, "Linear Transfer"=w116, "Linear Raw"=w109, "Saturation Transfer"=w110, "Saturation Raw"=w108, "TRF Gate Current"=w106) -> (w107:T7)
              n124 = local write "Graph Cluster"(w107) -> ()
              n125 = local write "Status Indicator"(TRUE) -> ()
              n126 = property on="Status Indicator" class="Bool (strict)"("BoolText.Text"="Measuring\nTransfer") -> ()  [unwired: 2 in, 2 out]
              n127 = local write "TRF Path"(w89) -> ()
              n128 = local write "LKG Path"(w85) -> ()
            }
            frame #1 {
              n129 = local read "Gated SMU4 is..."() -> (w187:bool)
              n130 = case shown="True" w187 {
                frame False {
                }
                frame True {
                  n131 = local read "Light Bathe Cluster"() -> (w191:T2)
                  n132 = Unbundle By Name(w191) -> ("TG to BG:"=w190:bool, "TG to BG Durration"=w189:dbl)
                  n133 = local read "VISA resource name"() -> (w188:refnum<visa-resource-name>)
                  n134 = case shown="True" w190 {
                    tunnel: w189 -> [_ w193]
                    tunnel: w188 -> [_ w192]
                    frame False {
                    }
                    frame True {
                      n135 = flat-sequence {
                        tunnel: w192 -> [w194]
                        tunnel: w193 -> [w196]
                        tunnel: w192 -> [w197]
                        frame #0 {
                          w195 = u32 1 items=["positive pulse  ", "negative pulse  ", "level high  ", "level low  "] ("trigger signal")
                          n136 = call "HP415xA Op-Trigger Output.vi"("trigger signal"=w195, "VISA session"=w194) -> ()  [unwired: 2 in, 1 out]
                        }
                        frame #1 {
                          n137 = call "Time Delay"("Delay Time (s)"=w196) -> ()  [unwired: 10 in, 1 out]
                        }
                        frame #2 {
                          w198 = u32 0 items=["positive pulse  ", "negative pulse  ", "level high  ", "level low  "] ("trigger signal")
                          n138 = call "HP415xA Op-Trigger Output.vi"("trigger signal"=w198, "VISA session"=w197) -> ()  [unwired: 2 in, 1 out]
                        }
                      }
                    }
                  }
                }
              }
            }
            frame #2 {
              n139 = local read "Gated SMU4 is..."() -> (w199:bool)
              n140 = case shown="True" w199 {
                tunnel: w200 -> [_ w267]
                frame False {
                }
                frame True {
                  w244 = 0
                  w250 = 0
                  w293 = "XXX"
                  w296 = "XXX"
                  # "Transfer w/ Gated SMU4"
                  n141 = local write "Status Indicator"(TRUE) -> ()
                  n142 = property on="Saturation Transfer" class="XYGraph (strict)"("Active Plot"=0, "Plot.YScaleIdx"=0, "Active Plot"=1, "Plot.YScaleIdx"=0) -> ()  [unwired: 2 in, 2 out]
                  n143 = local read "Saved Folder:"() -> (w231:path)
                  n144 = local read "Saved Folder:"() -> (w237:path)
                  n145 = local read "Sample Properties:"() -> (w209:T9)
                  n146 = Build Path(base path=w231, name or relative path="TRF_SMU4") -> (appended path=w286:path)
                  n147 = property on="Status Indicator" class="Bool (strict)"("BoolText.Text"="Measuring\nTransfer (SMU4)") -> ()  [unwired: 2 in, 2 out]
                  n148 = Build Path(base path=w237, name or relative path="TRF") -> (appended path=w235:path)
                  n149 = Build Path(base path=w231, name or relative path="LKG") -> (appended path=w227:path)
                  n150 = Unbundle By Name(w209) -> ("Comments"=w217:string)
                  n151 = call <vilib>:"Check if File or Folder Exists.vi"("path"=w286) -> ("file or folder exists?"=w288:bool, "dup path"=w287:path)  [unwired: 8 in, 1 out]
                  n152 = local read "TG Dielectric Prop"() -> (w214:T1)
                  n153 = case shown="False" w288 {
                    tunnel: w287 -> [w319 w320]
                    tunnel: [w318 w320] -> w285
                    frame False {
                      n154 = Create Folder(path (use dialog)=w319) -> (created path=w318:path)  [unwired: 2 in, 2 out]
                    }
                    frame True {
                    }
                  }
                  n155 = Concatenate Strings(w217, "Gated SMU4" ("string")) -> (w215:string)
                  n156 = call <vilib>:"Check if File or Folder Exists.vi"("path"=w227) -> ("file or folder exists?"=w228:bool, "dup path"=w229:path)  [unwired: 8 in, 1 out]
                  n157 = call <vilib>:"Check if File or Folder Exists.vi"("path"=w235) -> ("file or folder exists?"=w233:bool, "dup path"=w234:path)  [unwired: 8 in, 1 out]
                  n158 = case shown="False" w228 {
                    tunnel: w229 -> [w313 w314]
                    tunnel: [w312 w314] -> w220
                    frame False {
                      n159 = Create Folder(path (use dialog)=w313) -> (created path=w312:path)  [unwired: 2 in, 2 out]
                    }
                    frame True {
                    }
                  }
                  n160 = Unbundle By Name(w214) -> ("Dielectric Constant (TG)"=w213:dbl, "Dielectric (d) (TG)"=w210:string)
                  n161 = case shown="False" w233 {
                    tunnel: w234 -> [w316 w317]
                    tunnel: [w315 w317] -> _
                    frame False {
                      n162 = Create Folder(path (use dialog)=w316) -> (created path=w315:path)  [unwired: 2 in, 2 out]
                    }
                    frame True {
                    }
                  }
                  n163 = Bundle By Name(cluster=w209, "Comments"=w215) -> (w212:T9)
                  n164 = Bundle By Name(cluster=w212, "Dielectric (d)"=w210) -> (w211:T9)
                  n165 = Unbundle(w212) -> ("Index (#)"=w302:string, "Index (ABC)"=w301:string, "Length"=w290:string, "Width"=w292:string, "T (K)"=w269:dbl)  [unwired: 9 out]
                  n166 = Concatenate Strings(w302, w301) -> (w224:string)
                  n167 = Decimal String To Number(string=w290) -> (number=w299:i32)  [unwired: 2 in, 1 out]
                  n168 = Decimal String To Number(string=w292) -> (number=w298:i32)  [unwired: 2 in, 1 out]
                  n169 = Equal?(x=w290, y=w296) -> (x = y?=w297:bool)
                  n170 = Equal?(x=w292, y=w293) -> (x = y?=w294:bool)
                  n171 = Number To Decimal String(number=w299) -> (decimal integer string=w295:string)  [unwired: 1 in]
                  n172 = Number To Decimal String(number=w298) -> (decimal integer string=w291:string)  [unwired: 1 in]
                  n173 = Select(t=w296, s=w297, f=w295) -> (s? t:f=w223:string)
                  n174 = Select(t=w293, s=w294, f=w291) -> (s? t:f=w222:string)
                  n175 = Number To Decimal String(number=w269) -> (decimal integer string=w221:string)  [unwired: 1 in]
                  n176 = call "Build Text3"("T"=w221, "Index"=w224, "Length"=w223, "Width"=w222) -> ("Result"=w225:string)  [unwired: 10 in, 1 out]
                  n177 = call "Build Text"("T"=w221, "Index"=w224, "Length"=w223, "Width"=w222) -> ("Result"=w305:string)  [unwired: 10 in, 1 out]
                  n178 = local read "TRF Cluster"() -> (w262:T10)
                  n179 = local read "Compliance Cluster"() -> (w272:T6)
                  n180 = Unbundle By Name(w262) -> ("Loop Step"=w265:dbl, "First Step"=w264:dbl)
                  n181 = Build Path(base path=w220, name or relative path=w225) -> (appended path=w226:path)
                  n182 = Build Path(base path=w285, name or relative path=w305) -> (appended path=w300:path)
                  n183 = Unbundle By Name(w272) -> ("Var1 sweep settings"=w270:T16, "Var2 step settings"=w271:T17)
                  n184 = Multiply(x=w265, y=w267) -> (x*y=w268:dbl)
                  n185 = local read "TRF Cluster"() -> (w277:T10)
                  n186 = local read "TRF Cluster"() -> (w280:T10)
                  n187 = call <vilib>:"Check if File or Folder Exists.vi"("path"=w226) -> ("file or folder exists?"=w203:bool, "dup path"=w204:path)  [unwired: 8 in, 1 out]
                  n188 = call <vilib>:"Check if File or Folder Exists.vi"("path"=w300) -> ("file or folder exists?"=w207:bool, "dup path"=w206:path)  [unwired: 8 in, 1 out]
                  n189 = local read "Gate Current Cluster"() -> (w219:T3)
                  n190 = Unbundle By Name(w280) -> ("Start 4"=w279:dbl, "Total Points 2"=w278:u16)
                  n191 = local read "TRF Cluster"() -> (w273:T10)
                  n192 = Unbundle By Name(w277) -> ("Start 3"=w276:dbl, "Stop 2"=w275:dbl, "Step 3"=w274:dbl)
                  n193 = Unbundle(w271) -> ("compliance (A)"=w307:dbl, "compliance (V)"=w306:dbl)
                  n194 = Add(x=w264, y=w268) -> (x+y=w263:dbl)
                  n195 = Unbundle(w270) -> ("sweep spacing (linear: 0)"=w311:u16, "sweep mode"=w310:bool, "compliance (V)"=w309:dbl, "compliance (A)"=w308:dbl)
                  n196 = call "Add_File_NumExt.vi"("Extension"=".TRF" ("string"), "file or folder exists?"=w207, "Path In"=w206) -> ("Path Out"=w205:path)  [unwired: 8 in]
                  n197 = call "Add_File_NumExt.vi"("Extension"=".LKG" ("string"), "file or folder exists?"=w203, "Path In"=w204) -> ("Path Out"=w201:path)  [unwired: 8 in]
                  n198 = local read "VISA resource name"() -> (w261:refnum<visa-resource-name>)
                  n199 = Unbundle By Name(w273) -> ("Integration Time 3"=w258:u32)
                  n200 = Unbundle By Name(w219) -> ("Gate Current (TRF)"=w218:T18)
                  n201 = Bundle("Start 3"=w276, "Stop 2"=w275, "Step 3"=w274, "sweep spacing (linear: 0)"=w311, "sweep mode"=w310, "compliance (V)"=w309, "compliance (A)"=w308) -> (w260:T19)  [unwired: 1 in]
                  n202 = Bundle By Name(cluster=w262, "Step 4"=w263) -> (w266:T10)
                  n203 = Bundle("compliance (A)"=w307, "compliance (V)"=w306, "Start 4"=w279, "Total Points 2"=w278, w263) -> (w259:T20)  [unwired: 1 in]
                  n204 = call "transfer char run_subvi_SMU4_14_05_22_JWa.vi"("VISA session"=w261, "Y2 axis settings"=w218, "LKG Path"=w201, "Var1 sweep settings"=w260, "Var2 step settings"=w259, "integration time"=w258, "Input Path"=w205, "Dielectric Constant"=w213, "Sample Properties:"=w211) -> ("Check Cluster"=w255:T21, "Output"=w256:T22, "Graph Cluster"=w254:T23, "error?"=w257:errorcluster)  [unwired: 3 in]
                  n205 = local write "TRF Cluster"(w266) -> ()
                  n206 = local write "LKG Path"(w201) -> ()
                  n207 = local write "TRF Path"(w205) -> ()
                  n208 = local write "Vt Cluster"(w255) -> ()
                  n209 = local write "Char Cluster"(w256) -> ()
                  n210 = Unbundle By Name(w254) -> ("Linear Sqrt"=w252:cluster{dbl[], "trace":dbl[]}[], "Linear Log"=w251:cluster{dbl[], "trace":dbl[]}[], "Linear Raw"=w240:cluster{dbl[], dbl[]}[], "Saturation Sqrt"=w243:cluster{dbl[], "trace":dbl[]}[], "Saturation Log"=w242:cluster{dbl[], "trace":dbl[]}[], "Saturation Raw"=w239:cluster{dbl[], "trace":dbl[]}[], "Gate Current"=w232:cluster{dbl[], "trace":dbl[]}[])
                  n211 = local write "error out"(w257) -> ()
                  n212 = local read "Graph Cluster"() -> (w253:T7)
                  n213 = Index Array(array=w252, index=w250) -> (element=w249:cluster{dbl[], "trace":dbl[]})
                  n214 = Index Array(array=w251, index=w250) -> (element=w248:cluster{dbl[], "trace":dbl[]})
                  n215 = Index Array(array=w243, index=w244) -> (element=w245:cluster{dbl[], "trace":dbl[]})
                  n216 = Index Array(array=w242, index=w244) -> (element=w246:cluster{dbl[], "trace":dbl[]})
                  n217 = Build Array(w249, w248) -> (w247:cluster{dbl[], "trace":dbl[]}[])
                  n218 = Build Array(w245, w246) -> (w241:cluster{dbl[], "trace":dbl[]}[])
                  n219 = Bundle By Name(cluster=w253, "Linear Transfer"=w247, "Linear Raw"=w240, "Saturation Transfer"=w241, "Saturation Raw"=w239, "TRF Gate Current"=w232) -> (w238:T7)
                  n220 = local write "Graph Cluster"(w238) -> ()
                }
              }
            }
          }
        }
      }
    }
    frame #2 {
      n221 = local write "Status Indicator"(FALSE) -> ()
    }
    frame #3 {
      # "This frame creates the countdown timer for the wait inbetween the\nTransfer and Transport (if both selected)."
      n222 = disable-structure shown="Disabled" {
        frame Disabled {
          n223 = node-c288(1) -> (w335:T13)  [unwired: 1 in]
          n224 = timed-loop {
            timing: w335 -> [_]
            timing-out: [_] -> w334
            i -> [w346]
            stop <- w347 stop-if-true
            n225 = node-c288() -> ()  [unwired: 1 in, 1 out]
            n226 = local read "TRF Cluster"() -> (w340:T10)
            n227 = local read "TSP Cluster"() -> (w341:T11)
            n228 = local read "Wait Cluster"() -> (w339:T5)
            n229 = Unbundle By Name(w340) -> ("Transfer 2"=w343:bool)
            n230 = Unbundle By Name(w341) -> ("Transport"=w342:bool)
            n231 = Unbundle By Name(w339) -> ("Wait Time (s)"=w337:dbl)
            n232 = And(x=w343, y=w342) -> (x .and. y?=w351:bool)
            n233 = Select(t=w337, s=w351, f=0) -> (s? t:f=w349:dbl)
            n234 = Multiply(x=w346, y=0.001) -> (x*y=w344:dbl)
            n235 = Subtract(x=w349, y=w344) -> (x-y=w338:dbl)
            n236 = Select(t="Waiting...", s=w351, f="Ready") -> (s? t:f=w353:string)
            n237 = property on="Status Indicator" class="Bool (strict)"("BoolText.Text"=w353) -> ()  [unwired: 2 in, 2 out]
            n238 = Bundle("Wait Time (s)"=w337, w338) -> (w336:cluster{"Wait Time (s)":dbl, dbl})  [unwired: 1 in]
            n239 = Less Or Equal?(x=w338, y=0) -> (x <= y?=w347:bool)
            n240 = local write "Wait Cluster"(w336) -> ()
            n241 = node-c288() -> ()  [unwired: 1 in, 1 out]
          }
          n242 = node-c288(w334) -> ()  [unwired: 1 out]
        }
        frame Enabled {
        }
      }
      n243 = local read "Light Bathe Cluster"() -> (w322:T2)
      n244 = Unbundle By Name(w322) -> ("TRF to TSP:"=w325:bool, "TRF to TSP Duration"=w324:dbl)
      n245 = local read "VISA resource name"() -> (w323:refnum<visa-resource-name>)
      n246 = case shown="True" w325 {
        tunnel: w324 -> [_ w327]
        tunnel: w323 -> [_ w326]
        frame False {
        }
        frame True {
          n247 = flat-sequence {
            tunnel: w326 -> [w328]
            tunnel: w327 -> [w330]
            tunnel: w326 -> [w331]
            frame #0 {
              w329 = u32 1 items=["positive pulse  ", "negative pulse  ", "level high  ", "level low  "] ("trigger signal")
              n248 = call "HP415xA Op-Trigger Output.vi"("trigger signal"=w329, "VISA session"=w328) -> ()  [unwired: 2 in, 1 out]
            }
            frame #1 {
              n249 = call "Time Delay2"("Delay Time (s)"=w330) -> ()  [unwired: 10 in, 1 out]
            }
            frame #2 {
              w332 = u32 0 items=["positive pulse  ", "negative pulse  ", "level high  ", "level low  "] ("trigger signal")
              n250 = call "HP415xA Op-Trigger Output.vi"("trigger signal"=w332, "VISA session"=w331) -> ()  [unwired: 2 in, 1 out]
            }
          }
        }
      }
    }
    frame #4 {
      n251 = local read "TSP Cluster"() -> (w362:T11)
      n252 = Unbundle By Name(w362) -> ("Transport"=w361:bool)
      n253 = case shown="True" w361 {
        frame False {
        }
        frame True {
          n254 = stacked-sequence {
            frame #0 {
              w396 = "XXX"
              w400 = "XXX"
              # "TSP w/o SMU4"
              n255 = local read "Saved Folder:"() -> (w376:path)
              n256 = property on="Status Indicator" class="Bool (strict)"("BoolText.Text"="Measuring\nTransport") -> ()  [unwired: 2 in, 2 out]
              n257 = local read "Sample Properties:"() -> (w412:T9)
              n258 = Build Path(base path=w376, name or relative path="TSP") -> (appended path=w389:path)
              n259 = Unbundle(w412) -> ("Index (#)"=w411:string, "Index (ABC)"=w410:string, "Length"=w401:string, "Width"=w397:string, "T (K)"=w371:dbl)  [unwired: 9 out]
              n260 = Concatenate Strings(w411, w410) -> (w409:string)
              n261 = Decimal String To Number(string=w401) -> (number=w404:i32)  [unwired: 2 in, 1 out]
              n262 = Decimal String To Number(string=w397) -> (number=w403:i32)  [unwired: 2 in, 1 out]
              n263 = call <vilib>:"Check if File or Folder Exists.vi"("path"=w389) -> ("file or folder exists?"=w391:bool, "dup path"=w390:path)  [unwired: 8 in, 1 out]
              n264 = case shown="False" w391 {
                tunnel: w390 -> [w425 w426]
                tunnel: [w424 w426] -> w388
                frame False {
                  n265 = Create Folder(path (use dialog)=w425) -> (created path=w424:path)  [unwired: 2 in, 2 out]
                }
                frame True {
                }
              }
              n266 = Equal?(x=w400, y=w401) -> (x = y?=w402:bool)
              n267 = Equal?(x=w396, y=w397) -> (x = y?=w405:bool)
              n268 = Number To Decimal String(number=w404) -> (decimal integer string=w399:string)  [unwired: 1 in]
              n269 = Number To Decimal String(number=w403) -> (decimal integer string=w395:string)  [unwired: 1 in]
              n270 = Select(t=w400, s=w402, f=w399) -> (s? t:f=w398:string)
              n271 = Select(t=w396, s=w405, f=w395) -> (s? t:f=w394:string)
              n272 = call "Build Text2"("T"=w371, "Index"=w409, "Length"=w398, "Width"=w394) -> ("Result"=w393:string)  [unwired: 10 in, 1 out]
              n273 = local read "Compliance Cluster"() -> (w375:T6)
              n274 = Build Path(base path=w388, name or relative path=w393) -> (appended path=w406:path)
              n275 = Unbundle By Name(w375) -> ("Var1 sweep settings 2"=w374:T16, "Var2 step settings 2"=w373:T17)
              n276 = local read "TSP Cluster"() -> (w387:T11)
              n277 = local read "TSP Cluster"() -> (w378:T11)
              n278 = call <vilib>:"Check if File or Folder Exists.vi"("path"=w406) -> ("file or folder exists?"=w408:bool, "dup path"=w407:path)  [unwired: 8 in, 1 out]
              n279 = local read "Gate Current Cluster"() -> (w365:T3)
              n280 = Unbundle By Name(w378) -> ("Start"=w383:dbl, "Total Points"=w382:u16, "Step"=w381:dbl)
              n281 = local read "TSP Cluster"() -> (w380:T11)
              n282 = Unbundle By Name(w387) -> ("Start 2"=w386:dbl, "Stop 3"=w385:dbl, "Step 2"=w384:dbl)
              n283 = Unbundle(w373) -> ("compliance (A)"=w418:dbl, "compliance (V)"=w417:dbl)
              n284 = Unbundle(w374) -> ("sweep spacing (linear: 0)"=w423:u16, "sweep mode"=w422:bool, "compliance (V)"=w421:dbl, "compliance (A)"=w420:dbl)
              n285 = call "Add_File_NumExt.vi"("Extension"=".TSP" ("string"), "file or folder exists?"=w408, "Path In"=w407) -> ("Path Out"=w372:path)  [unwired: 8 in]
              n286 = local read "VISA resource name"() -> (w377:refnum<visa-resource-name>)
              n287 = Unbundle By Name(w365) -> ("Gate Current (TSP)"=w364:T18)
              n288 = Unbundle By Name(w380) -> ("Integration Time"=w379:u32)
              n289 = Bundle("Start 2"=w386, "Stop 3"=w385, "Step 2"=w384, "sweep spacing (linear: 0)"=w423, "sweep mode"=w422, "compliance (V)"=w421, "compliance (A)"=w420) -> (w419:T24)  [unwired: 1 in]
              n290 = Bundle("compliance (A)"=w418, "compliance (V)"=w417, "Start"=w383, "Total Points"=w382, "Step"=w381) -> (w416:T25)  [unwired: 1 in]
              n291 = local write "TSP Path"(w372) -> ()
              n292 = call "transport char run_subvi_2014_05_30_JWa.vi"("VISA session"=w377, "Y2 axis settings"=w364, "Var1 sweep settings"=w419, "Var2 step settings"=w416, "integration time"=w379, "Path"=w372, "Sample Properties:"=w412) -> ("Graph Cluster"=w370:T26, "error?"=w415:errorcluster)  [unwired: 6 in, 1 out]
              n293 = local write "error out"(w415) -> ()
              n294 = Unbundle By Name(w370) -> ("Transport"=w367:cluster{dbl[], dbl[]}[], "Gate Current"=w366:cluster{dbl[], dbl[]}[])
              n295 = local read "Graph Cluster"() -> (w369:T7)
              n296 = Bundle By Name(cluster=w369, "Transport"=w367, "TSP Gate Current"=w366) -> (w368:T7)
              n297 = local write "Graph Cluster"(w368) -> ()
              n298 = local write "Status Indicator"(TRUE) -> ()
            }
            frame #1 {
              n299 = local read "Gated SMU4 is..."() -> (w427:bool)
              n300 = case shown="True" w427 {
                frame False {
                }
                frame True {
                  n301 = local read "Light Bathe Cluster"() -> (w431:T2)
                  n302 = Unbundle By Name(w431) -> ("TG to BG (TSP):"=w430:bool, "TG to BG Durration 3"=w429:dbl)
                  n303 = local read "VISA resource name"() -> (w428:refnum<visa-resource-name>)
                  n304 = case shown="True" w430 {
                    tunnel: w429 -> [_ w433]
                    tunnel: w428 -> [_ w432]
                    frame False {
                    }
                    frame True {
                      n305 = flat-sequence {
                        tunnel: w432 -> [w434]
                        tunnel: w433 -> [w436]
                        tunnel: w432 -> [w437]
                        frame #0 {
                          w435 = u32 1 items=["positive pulse  ", "negative pulse  ", "level high  ", "level low  "] ("trigger signal")
                          n306 = call "HP415xA Op-Trigger Output.vi"("trigger signal"=w435, "VISA session"=w434) -> ()  [unwired: 2 in, 1 out]
                        }
                        frame #1 {
                          n307 = call "Time Delay3"("Delay Time (s)"=w436) -> ()  [unwired: 10 in, 1 out]
                        }
                        frame #2 {
                          w438 = u32 0 items=["positive pulse  ", "negative pulse  ", "level high  ", "level low  "] ("trigger signal")
                          n308 = call "HP415xA Op-Trigger Output.vi"("trigger signal"=w438, "VISA session"=w437) -> ()  [unwired: 2 in, 1 out]
                        }
                      }
                    }
                  }
                }
              }
            }
            frame #2 {
              # "TSP w/ SMU4"
              n309 = local read "Gated SMU4 is..."() -> (w439:bool)
              n310 = case shown="True" w439 {
                frame False {
                }
                frame True {
                  w475 = "XXX"
                  w479 = "XXX"
                  n311 = local write "Status Indicator"(TRUE) -> ()
                  n312 = local read "Saved Folder:"() -> (w455:path)
                  n313 = local read "TSP Cluster"() -> (w459:T11)
                  n314 = local read "Sample Properties:"() -> (w489:T9)
                  n315 = property on="Status Indicator" class="Bool (strict)"("BoolText.Text"="     Measuring\nTransport SMU4") -> ()  [unwired: 2 in, 2 out]
                  n316 = Unbundle By Name(w459) -> ("Integration Time"=w458:u32)
                  n317 = Build Path(base path=w455, name or relative path="TSP_SMU4") -> (appended path=w468:path)
                  n318 = call <vilib>:"Check if File or Folder Exists.vi"("path"=w468) -> ("file or folder exists?"=w470:bool, "dup path"=w469:path)  [unwired: 8 in, 1 out]
                  n319 = Unbundle(w489) -> ("Index (#)"=w488:string, "Index (ABC)"=w487:string, "Length"=w480:string, "Width"=w476:string, "T (K)"=w451:dbl)  [unwired: 9 out]
                  n320 = case shown="False" w470 {
                    tunnel: w469 -> [w502 w503]
                    tunnel: [w501 w503] -> w467
                    frame False {
                      n321 = Create Folder(path (use dialog)=w502) -> (created path=w501:path)  [unwired: 2 in, 2 out]
                    }
                    frame True {
                    }
                  }
                  n322 = Concatenate Strings(w488, w487) -> (w486:string)
                  n323 = Decimal String To Number(string=w480) -> (number=w483:i32)  [unwired: 2 in, 1 out]
                  n324 = Decimal String To Number(string=w476) -> (number=w482:i32)  [unwired: 2 in, 1 out]
                  n325 = Equal?(x=w479, y=w480) -> (x = y?=w481:bool)
                  n326 = Equal?(x=w475, y=w476) -> (x = y?=w484:bool)
                  n327 = Number To Decimal String(number=w483) -> (decimal integer string=w478:string)  [unwired: 1 in]
                  n328 = Number To Decimal String(number=w482) -> (decimal integer string=w474:string)  [unwired: 1 in]
                  n329 = Select(t=w479, s=w481, f=w478) -> (s? t:f=w477:string)
                  n330 = Select(t=w475, s=w484, f=w474) -> (s? t:f=w473:string)
                  n331 = call "Build Text6"("T"=w451, "Index"=w486, "Length"=w477, "Width"=w473) -> ("Result"=w472:string)  [unwired: 10 in, 1 out]
                  n332 = local read "Compliance Cluster"() -> (w454:T6)
                  n333 = Build Path(base path=w467, name or relative path=w472) -> (appended path=w485:path)
                  n334 = Unbundle By Name(w454) -> ("Var1 sweep settings 2"=w453:T16, "Var2 step settings 2"=w452:T17)
                  n335 = local read "TSP Cluster"() -> (w466:T11)
                  n336 = local read "TSP Cluster"() -> (w457:T11)
                  n337 = call <vilib>:"Check if File or Folder Exists.vi"("path"=w485) -> ("file or folder exists?"=w441:bool, "dup path"=w442:path)  [unwired: 8 in, 1 out]
                  n338 = local read "Gate Current Cluster"() -> (w445:T3)
                  n339 = Unbundle By Name(w457) -> ("Start"=w462:dbl, "Total Points"=w461:u16, "Step"=w460:dbl)
                  n340 = Unbundle By Name(w466) -> ("Start 2"=w465:dbl, "Stop 3"=w464:dbl, "Step 2"=w463:dbl)
                  n341 = Unbundle(w452) -> ("compliance (A)"=w495:dbl, "compliance (V)"=w494:dbl)
                  n342 = call "Add_File_NumExt.vi"("Extension"=".TSP" ("string"), "file or folder exists?"=w441, "Path In"=w442) -> ("Path Out"=w440:path)  [unwired: 8 in]
                  n343 = Unbundle(w453) -> ("sweep spacing (linear: 0)"=w500:u16, "sweep mode"=w499:bool, "compliance (V)"=w498:dbl, "compliance (A)"=w497:dbl)
                  n344 = local read "VISA resource name"() -> (w456:refnum<visa-resource-name>)
                  n345 = Unbundle By Name(w445) -> ("Gate Current (TSP)"=w444:T18)
                  n346 = Bundle("Start 2"=w465, "Stop 3"=w464, "Step 2"=w463, "sweep spacing (linear: 0)"=w500, "sweep mode"=w499, "compliance (V)"=w498, "compliance (A)"=w497) -> (w496:T24)  [unwired: 1 in]
                  n347 = Bundle("compliance (A)"=w495, "compliance (V)"=w494, "Start"=w462, "Total Points"=w461, "Step"=w460) -> (w493:T25)  [unwired: 1 in]
                  n348 = local write "TSP Path"(w440) -> ()
                  n349 = call "transport char run_subvi_2014_05_29_SMU4_JWa.vi"("VISA session"=w456, "Y2 axis settings"=w444, "Var1 sweep settings"=w496, "Var2 step settings"=w493, "integration time"=w458, "Path"=w440, "Sample Properties:"=w489) -> ("Graph Cluster"=w450:T26, "error?"=w492:errorcluster)  [unwired: 6 in, 1 out]
                  n350 = local read "Graph Cluster"() -> (w449:T7)
                  n351 = local write "error out"(w492) -> ()
                  n352 = Unbundle By Name(w450) -> ("Transport"=w447:cluster{dbl[], dbl[]}[], "Gate Current"=w446:cluster{dbl[], dbl[]}[])
                  n353 = Bundle By Name(cluster=w449, "Transport"=w447, "TSP Gate Current"=w446) -> (w448:T7)
                  n354 = local write "Graph Cluster"(w448) -> ()
                }
              }
            }
          }
        }
      }
    }
    frame #5 {
      n355 = local write "Status Indicator"(FALSE) -> ()
      n356 = property on="Status Indicator" class="Bool (strict)"("BoolText.Text"="Ready") -> ()  [unwired: 2 in, 2 out]
    }
    frame #6 {
      n357 = disable-structure shown="Disabled" {
        disable-tunnel: w507 -> [w509 _]
        disable-tunnel: w506 -> [w508 _]
        frame Disabled {
          n358 = node-c288(100) -> (w514:T13)  [unwired: 3 in]
          n359 = timed-loop {
            timing: w514 -> [_]
            timing-out: [_] -> w513
            tunnel: w509 -> [w525]
            tunnel: w508 -> [w524]
            tunnel: ["Stop \nCountdown"] -> _
            i -> [w530]
            stop <- w520 stop-if-true
            n360 = node-c288() -> ()  [unwired: 1 in, 1 out]
            n361 = local read "TRF Cluster"() -> (w519:T10)
            n362 = Unbundle By Name(w519) -> ("Loop Wait"=w517:dbl)
            n363 = Equal?(x=w524, y=w525) -> (x = y?=w526:bool)
            n364 = Select(t=0, s=w526, f=w517) -> (s? t:f=w522:dbl)
            n365 = Multiply(x=0.1, y=w530) -> (x*y=w528:dbl)
            n366 = Subtract(x=w522, y=w528) -> (x-y=w516:dbl)
            n367 = Less Or Equal To 0?(x=w516) -> (x <= 0?=w521:bool)
            n368 = Bundle("Loop Wait"=w517, w516) -> (w518:cluster{"Loop Wait":dbl, dbl})  [unwired: 1 in]
            n369 = property on="Status Indicator" class="Bool (strict)"("BoolText.Text"="Waiting...") -> ()  [unwired: 2 in, 2 out]
            n370 = local write "Wait Cluster"(w518) -> ()
            n371 = Or(x=w521, y="Stop \nCountdown") -> (x .or. y?=w520:bool)
            n372 = node-c288() -> ()  [unwired: 1 in, 1 out]
          }
          n373 = node-c288(w513) -> (w510:errorcluster)
          n374 = property on="Status Indicator" class="Bool (strict)"(error in=w510, "BoolText.Text"="Ready") -> ()  [unwired: 1 in, 2 out]
        }
        frame Enabled {
        }
      }
    }
  }
  n375 = local write "VISA resource name out"(w6) -> ()
